vi "Example3.vi"() -> ()   [LabVIEW 2019]
uses:
  source code/Container/dotNET Container/dotNET Container.lvclass
  D:/Namratha/MDI/LabVIEW-MDI-develop_LV2019/source code/Container/Container base/Container base.lvclass
  source code/Document/LV Doc/Child/LV DEV/LV DEV.lvclass
  D:/Namratha/MDI/LabVIEW-MDI-develop_LV2019/source code/Document/Document base/Document.lvclass
  source code/Document/Py Doc/Child Classes/Py Editor/Py Editor.lvclass
  source code/Document/Py Doc/Child Classes/Py Shell/Py Shell.lvclass
  source code/MDI Library/Public/Create.vi
  source code/Document/LV Doc/Child/LV DEV/public/LV Dev Doc - Instantiate with Path.vi
  source code/Document/LV Doc/Child/LV DEV/public/LV Dev Doc - Instantiate with Ref.vi
  source code/MDI Library/Public/Add.vi
  source code/MDI Library/Public/Show.vi
  source code/MDI Library/Public/Tile.vi
  source code/MDI Library/Public/Cascade.vi
  source code/MDI Library/Public/Save.vi
  source code/MDI Library/Public/Load.vi
  source code/MDI Library/Public/Remove.vi
  source code/Document/Document base/Document.lvclass
  source code/MDI Library/LV MDI.lvclass
  source code/Document/Py Doc/Py Doc.lvclass
  System.Windows.Forms
panel:
  in  "LabVIEW Version":u16(ring) items=["LabVIEW 2019", "LabVIEW 2018", "LabVIEW 2016"]
  in  "Py File Path":path
  in  "Load":bool
  in  "XML File Path":path=path "C:/Users/namratha.balakrishna/Documents/Namratha/MDI.xml"
  in  "Save":bool
  in  "Cascade":bool
  in  "Tile":bool
  in  "Stop":bool
  in  "Show":bool
  in  "LV Doc Path":path
  in  "Panel Reference":refnum<k24>(container)
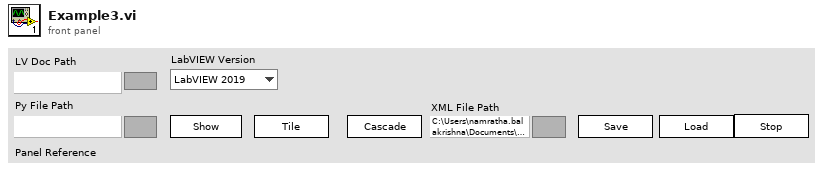
[diagram p1: front panel]
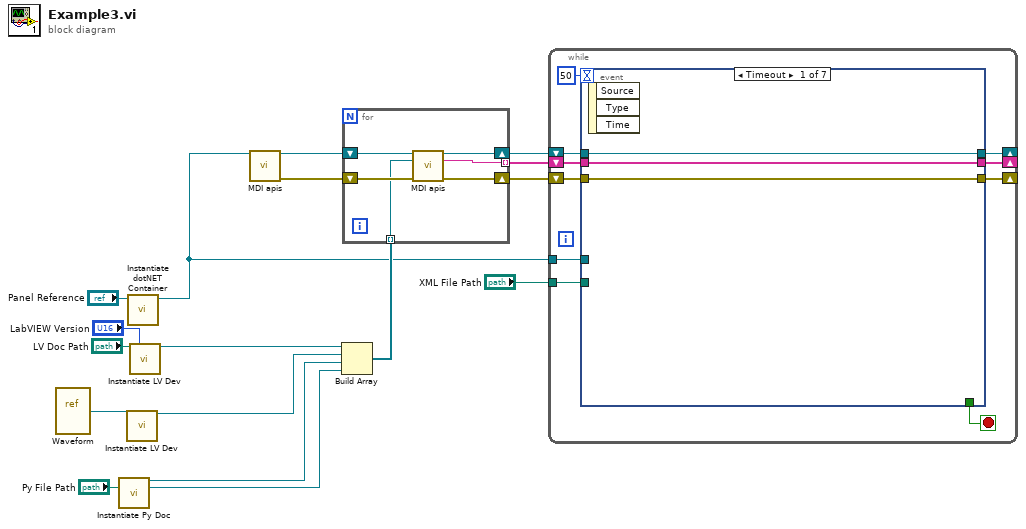
[diagram p0: block diagram]
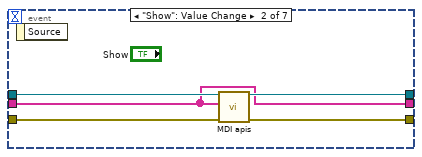
[diagram p2: hidden frame]
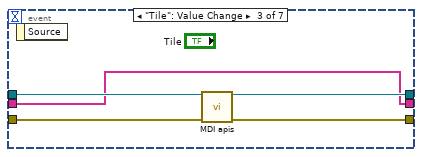
[diagram p3: hidden frame]
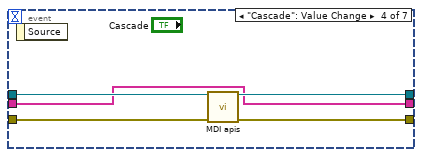
[diagram p4: hidden frame]
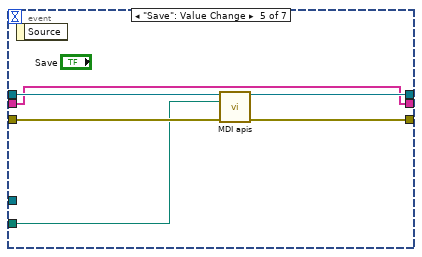
[diagram p5: hidden frame]
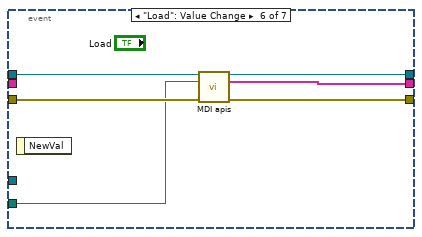
[diagram p6: hidden frame]
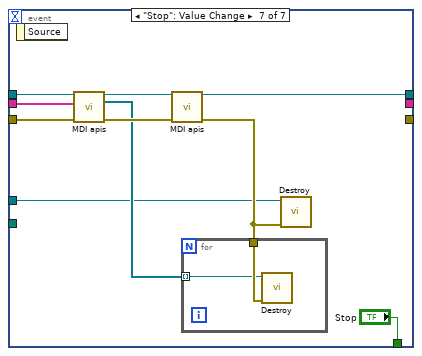
[diagram p7: hidden frame]
diagram:
  n1 = vi-ref "Waveform.vi"() -> (w2:refnum<vi>)
  n2 = call "Instantiate Py Doc.vi"("Py File Path"="Py File Path") -> ("Py Editor.lvclass"=w4:refnum<class "Py Editor.lvclass">, "Py Shell.lvclass"=w3:refnum<class "Py Shell.lvclass">)  [unwired: 12 in, 1 out]
  n3 = call-poly "Instantiate LV Dev.vi"("VI Refnum"=w2) -> ("LV DEV"=w12:refnum<class "LV DEV.lvclass">)  [unwired: 13 in, 1 out]
  n4 = call "Instantiate dotNET Container.vi"("Panel Reference"="Panel Reference") -> ("dotNET Container out"=w7:refnum<class "dotNET Container.lvclass">)  [unwired: 9 in, 1 out]
  n5 = call-poly "Instantiate LV Dev.vi"("LV Doc Path"="LV Doc Path", "LabVIEW Version"="LabVIEW Version") -> ("LV DEV"=w13:refnum<class "LV DEV.lvclass">)  [unwired: 12 in, 1 out]
  n6 = call-poly "MDI apis.vi"("Container"=w7) -> ("LV MDI"=w17:refnum<class "LV MDI.lvclass">, "error out"=w16:errorcluster)  [unwired: 13 in]
  n7 = Build Array(w13, w12, w4, w3) -> (w15:refnum<class "Document.lvclass">[])
  n8 = for {
    shift-right: [w21] -> w9
    shift-left: w17 -> [w23]
    shift-right: [w20] -> w10
    shift-left: w16 -> [w22]
    tunnel: w15 -> [w19] mode=indexing
    tunnel: [w18] -> w8 mode=indexing
    n9 = call-poly "MDI apis.vi"("LV MDI.lvclass"=w23, "Document class"=w19, "error in (no error)"=w22) -> ("LV MDI.lvclass"=w21:refnum<class "LV MDI.lvclass">, "Doc UID"=w18:string, "error out"=w20:errorcluster)  [unwired: 10 in]
  }
  n10 = while {
    shift-right: [w30] -> _
    shift-left: w10 -> [w31]
    shift-right: [w28] -> _
    shift-left: w9 -> [w29]
    tunnel: w7 -> [w26]
    tunnel: "XML File Path" -> [w25]
    shift-right: [w24] -> _
    shift-left: w8 -> [w27]
    stop <- w32 stop-if-true
    n11 = event shown="[0] Timeout" {
      selector: _ -> [_ _ _ _ _ _ _]
      dyn-events: _ -> [_ _ _ _ _ _ _]
      timeout: 50 -> [_ _ _ _ _ _ _]
      tunnel: [_ _ _ _ _ _ "Stop"] -> w32
      tunnel: w31 -> [w36 w41 w45 w49 w55 w63 w68]
      tunnel: [w36 w40 w44 w48 w54 w62 _] -> w30
      tunnel: w29 -> [w35 w39 w46 w51 w57 w61 w67]
      tunnel: [w35 w38 w43 w50 w56 w60 w66] -> w28
      tunnel: w27 -> [w34 w37 w42 w47 w52 _ w64]
      tunnel: w26 -> [_ _ _ _ _ _ w65]
      tunnel: w25 -> [_ _ _ _ w53 w59 _]
      tunnel: [w34 w37 w42 w47 w52 w58 _] -> w24
      event Timeout {
        n12 = event-data() -> ()  [unwired: 1 in, 3 out]
      }
      event "Show": Value Change {
        n13 = event-data() -> ()  [unwired: 1 in, 1 out]
        n14 = call-poly "MDI apis.vi"("LV MDI in"=w39, "Doc UID[]"=w37, "error in (no error)"=w41) -> ("LV MDI out"=w38:refnum<class "LV MDI.lvclass">, "error out"=w40:errorcluster)  [unwired: 11 in]
      }
      event "Tile": Value Change {
        n15 = event-data() -> ()  [unwired: 1 in, 1 out]
        n16 = call-poly "MDI apis.vi"("LV MDI.lvclass"=w46, "error in (no error)"=w45) -> ("LV MDI.lvclass"=w43:refnum<class "LV MDI.lvclass">, "error out"=w44:errorcluster)  [unwired: 12 in]
      }
      event "Cascade": Value Change {
        n17 = event-data() -> ()  [unwired: 1 in, 1 out]
        n18 = call-poly "MDI apis.vi"("LV MDI in"=w51, "error in (no error)"=w49) -> ("LV MDI out"=w50:refnum<class "LV MDI.lvclass">, "error out"=w48:errorcluster)  [unwired: 12 in]
      }
      event "Save": Value Change {
        n19 = event-data() -> ()  [unwired: 1 in, 1 out]
        n20 = call-poly "MDI apis.vi"("LV MDI in"=w57, "XML File Path"=w53, "error in (no error)"=w55) -> ("LV MDI out"=w56:refnum<class "LV MDI.lvclass">, "error out"=w54:errorcluster)  [unwired: 11 in]
      }
      event "Load": Value Change {
        n21 = event-data() -> ()  [unwired: 1 in, 1 out]
        n22 = call-poly "MDI apis.vi"("LV MDI in"=w61, "XML File Path"=w59, "error in (no error)"=w63) -> ("LV MDI out"=w60:refnum<class "LV MDI.lvclass">, "Doc UID[]"=w58:string[], "error out"=w62:errorcluster)  [unwired: 10 in]
      }
      event "Stop": Value Change {
        n23 = event-data() -> ()  [unwired: 1 in, 1 out]
        n24 = call-poly "MDI apis.vi"("LV MDI in"=w67, "Doc UID[]"=w64, "error in (no error)"=w68) -> ("LV MDI out"=w71:refnum<class "LV MDI.lvclass">, "Doc obj[]"=w69:refnum<class "Document.lvclass">[], "error out"=w70:errorcluster)  [unwired: 10 in]
        n25 = call-poly "MDI apis.vi"("LV MDI in"=w71, "error in (no error)"=w70) -> ("LV MDI out"=w66:refnum<class "LV MDI.lvclass">, "error out"=w72:errorcluster)  [unwired: 12 in]
        n26 = for {
          tunnel: w72 -> [w75]
          tunnel: w69 -> [w74] mode=indexing
          n27 = call-dynamic "Destroy.vi"("error in (no error)"=w75, "Document in"=w74) -> ()  [unwired: 8 in, 2 out]
        }
        n28 = call-dynamic "Destroy.vi"("error in (no error)"=w72, "dotNET Container in"=w65) -> ()  [unwired: 8 in, 2 out]
      }
    }
  }
